vi "rootlocus.vi"() -> ()   [LabVIEW 2019]
uses:
  <vilib>/addons/Control Design/_Model Construction/Data Typedefs.llb/CD Margin Data.ctl
  <vilib>/addons/Control Design/_Model Construction/Model Creation.llb/Model Creation SubVI/cd_Create Transfer Function Model.vi
  <vilib>/addons/Control Design/_Frequency Response Analysis/Frequency Response.llb/Frequency Response subVI/cd_Gain and Phase Margin (Transfer Function).vi
  <vilib>/addons/Control Design/_Frequency Response Analysis/Frequency Response.llb/Frequency Response subVI/cd_Nyquist (Transfer Function).vi
  <vilib>/addons/Control Design/_Dynamic Analysis/Dynamic Analysis.llb/Dynamic Analysis subVI/cd_Root Locus (Transfer Function).vi
  <vilib>/addons/Control Design/_Time Response Analysis/Time Response.llb/Time Response subVI/cd_Impulse Response (Transfer Function).vi
  <vilib>/addons/Control Design/_Utility/Model Viewer.llb/Model Viewer SubVI/cd_Draw Transfer Function Equation (TF).vi
  <vilib>/addons/Control Design/_Model Construction/NI_LinSys_Model Creation.lvlib
  <vilib>/addons/Control Design/_Utility/NI_CD_Model Viewer.lvlib
  <vilib>/addons/Control Design/_Time Response Analysis/NI_CD_Time Response.lvlib
  <vilib>/addons/Control Design/_Dynamic Analysis/NI_CD_Dynamic Analysis.lvlib
  <vilib>/addons/Control Design/_Frequency Response Analysis/NI_CD_Frequency Response.lvlib
  <vilib>/addons/Control Design/_Model Construction/NI_LinSys_Data Typedefs.lvlib
panel:
  out "Gain and Phase Margins":T1 {"Phase Margin" format="%#.4g"; "P.M. Frequency" format="%#.4g"; "Gain Margin" format="%#.4g"; "G.M. Frequency" format="%#.4g"}
  out "Phase Plot":cluster{"W":dbl[], "Phase":dbl[]}[](graph)
  out "Magnitude Plot":cluster{"W":dbl[], "Magnitude":dbl[]}[](graph)
  out "Nyquist Plot":cluster{"W":dbl[], "Magnitude":dbl[]}[](graph)
  out "Root Locus Graph":cluster{dbl[], dbl[]}[](graph)
  out "impulse response":cluster{"time":dbl[], dbl[]}[](graph)
  out "Equation 2":picture
  in  "Denominator 2":dbl[](array[numeric]) format="%#.5g"
  in  "Numerator 2":dbl[](array[numeric]) format="%#.5g"
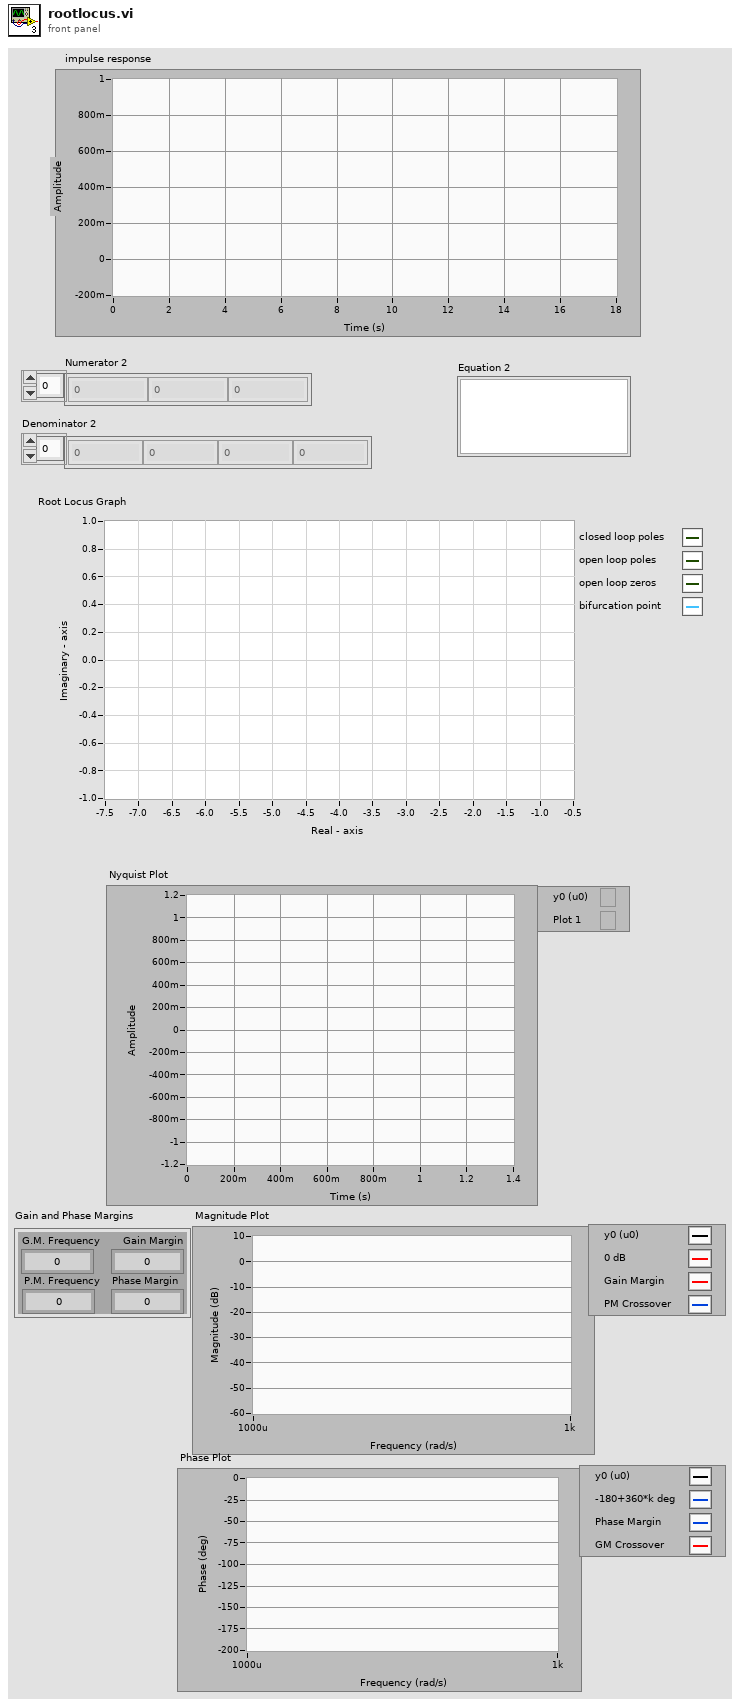
[diagram p1: front panel]
types:
  T1 = typedef "NI_LinSys_Data Typedefs.lvlib/CD Margin Data.ctl" = cluster{"G.M. Frequency":dbl, "Gain Margin":dbl, "P.M. Frequency":dbl, "Phase Margin":dbl}
  T2 = typedef "NI_LinSys_Model Typedefs.lvlib/CD Transfer Function Model (MIMO).ctl" = cluster{"properties":T3, "transfer function(s)":T4[][]}
  T3 = typedef "NI_LinSys_Model Typedefs.lvlib/CD General Elements.ctl" = cluster{"Model name":string, "Input names":string[], "Output names":string[], "Input Delays":dbl[], "Output Delays":dbl[], "Sampling Time":dbl, "Notes":string}
  T4 = typedef "NI_LinSys_Model Typedefs.lvlib/CD Transfer Function Model (SISO).ctl" = cluster{"Numerator":dbl[], "Denominator":dbl[], "delay":dbl}
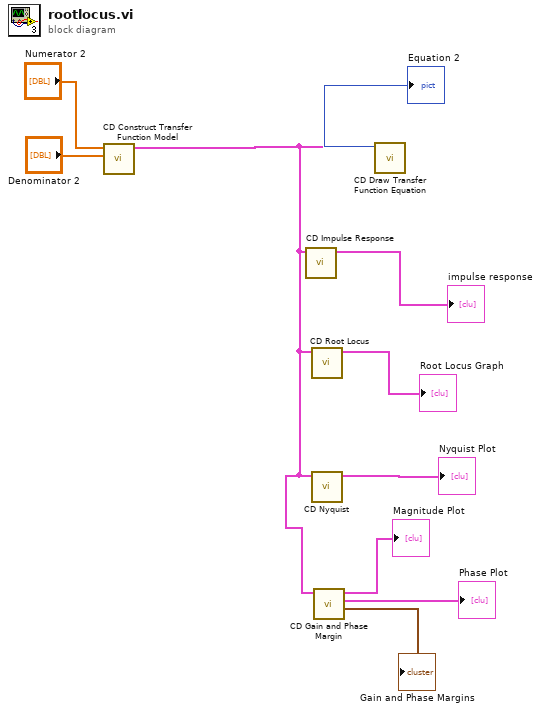
[diagram p0: block diagram]
diagram:
  n1 = call-poly <vilib>:"CD Construct Transfer Function Model.vi"("Denominator"="Denominator 2", "Numerator"="Numerator 2") -> ("Transfer Function Model"=w4:T2)  [unwired: 8 in, 1 out]
  n2 = call-poly <vilib>:"CD Impulse Response.vi"("Transfer Function Model"=w4) -> ("Impulse Response Graph"=→"impulse response":cluster{"time":dbl[], dbl[]}[])  [unwired: 8 in, 2 out]
  n3 = call-poly <vilib>:"CD Root Locus.vi"("Transfer Function Model"=w4) -> ("Root Locus Graph"=→"Root Locus Graph":cluster{dbl[], dbl[]}[])  [unwired: 7 in, 3 out]
  n4 = call-poly <vilib>:"CD Nyquist.vi"("Transfer Function Model"=w4) -> ("Nyquist Plot"=→"Nyquist Plot":cluster{"W":dbl[], "Magnitude":dbl[]}[])  [unwired: 8 in, 2 out]
  n5 = call-poly <vilib>:"CD Gain and Phase Margin.vi"("Transfer Function Model"=w4) -> ("Gain and Phase Margins"=→"Gain and Phase Margins":T1, "Phase Plot"=→"Phase Plot":cluster{"W":dbl[], "Phase":dbl[]}[], "Magnitude Plot"=→"Magnitude Plot":cluster{"W":dbl[], "Magnitude":dbl[]}[])  [unwired: 6 in, 2 out]
  n6 = call-poly <vilib>:"CD Draw Transfer Function Equation.vi"("Transfer Function Model"=w4) -> ("Equation"=→"Equation 2":picture)  [unwired: 8 in, 2 out]
